vi "Left Buttons.vi"(7 "Message type":string, 8 "error constant":errorcluster, 9 "Input":string) -> (0 "error out":errorcluster, 2 "Next State":T1, 4 "Pin Out":string, 5 "Msg":string)   [LabVIEW 2019, in "SubVI.lvlib"]
doc: "Performs functions set by left side buttons on the UI"
uses:
  SubVIs/SubVI.lvlib
  controls/State.ctl
  controls/Message Type.ctl
  controls/ATM Action.ctl
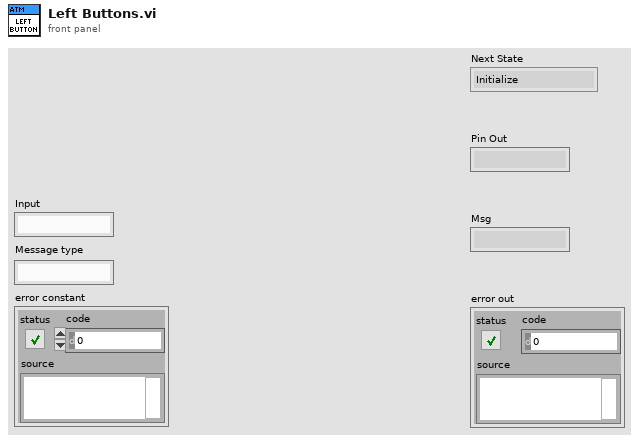
[diagram p1: front panel]
types:
  T1 = typedef "State.ctl" = enum16{"Initialize", "Wait for Event", "Terminate"}
  T2 = typedef "Message Type.ctl" = enum16{"Main Menu", "Balance", "Withdrawal Complete", "Deposit Complete", "Welcome", "Account", "Session", "Deposit", "Withdraw", "Failed"}
  T3 = typedef "ATM Action.ctl" = enum16{"User", "Deposit", "Withdraw"}
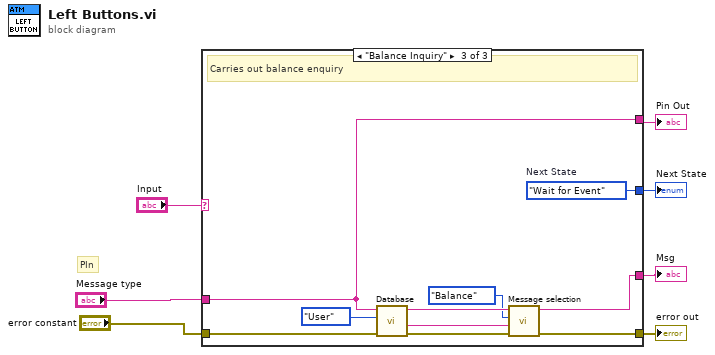
[diagram p0: block diagram]
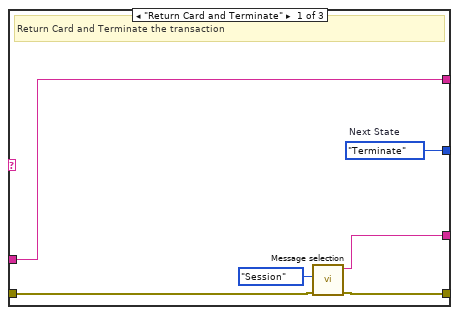
[diagram p2: hidden frame]
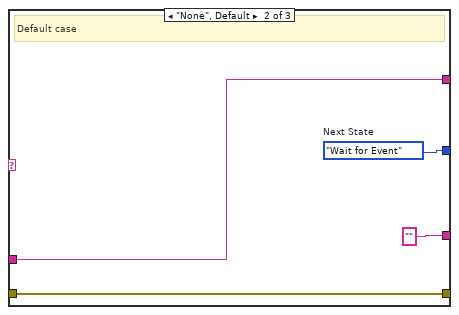
[diagram p3: hidden frame]
diagram:
  # "PIn"
  n1 = case shown="\"Balance Inquiry\"" "Input" {
    tunnel: "Message type" -> [w9 w15 w20]
    tunnel: [w13 "" ("Message Out") w21] -> w3
    tunnel: [w10 w17 w22] -> w2
    tunnel: "error constant" -> [w11 w17 w27]
    tunnel: [w9 w15 w20] -> w4
    tunnel: [w8 w14 w18] -> w1
    frame "Return Card and Terminate" {
      w8 = State."Terminate"  # Next State
      # "Return Card and Terminate the transaction"
      n2 = call "Message selection.vi"("error in (no error)"=w11, "state"=Message_Type."Session") -> ("error out"=w10:errorcluster, "Msg"=w13:string)  [unwired: 8 in]
    }
    frame "None", Default {
      w14 = State."Wait for Event"  # Next State
      # "Default case"
    }
    frame "Balance Inquiry" {
      w18 = State."Wait for Event"  # Next State
      # "Carries out balance enquiry"
      n3 = call "Database.vi"("error in"=w27, "Action"=ATM_Action."User", "User Input"=w20) -> ("error out"=w23:errorcluster, "Money Out"=w26:string, "Name"=w25:string)  [unwired: 5 in, 1 out]
      n4 = call "Message selection.vi"("error in (no error)"=w23, "Amount"=w26, "state"=Message_Type."Balance", "Message type"=w25) -> ("error out"=w22:errorcluster, "Msg"=w21:string)  [unwired: 6 in]
    }
  }
  "error out" <- w2
  "Msg" <- w3
  "Pin Out" <- w4
  "Next State" <- w1
